vi "Reset Manual Layout.vi"(8 "error in":errorcluster, 11 "Base Software in":refnum<class "Base Software.lvclass">) -> (0 "error out":errorcluster, 3 "Base Software out":refnum<class "Base Software.lvclass">)   [LabVIEW 2019, in "Base Software.lvlib" / "Main.lvlib" / "Base Software.lvclass"]
uses:
  Project/Base Software.lvclass
  Custom Controls/g_Identifiers.vi
  builds/Engine/Engine.lvlibp/Engine Messages/Reset Manual Layout Msg/Reset Manual Layout Msg.lvclass
  builds/Engine/Engine.lvlibp/Project/Engine.lvclass
  C:/Users/Public/Documents/Development/builds/Engine/Engine.lvlibp/Project/Engine.lvclass
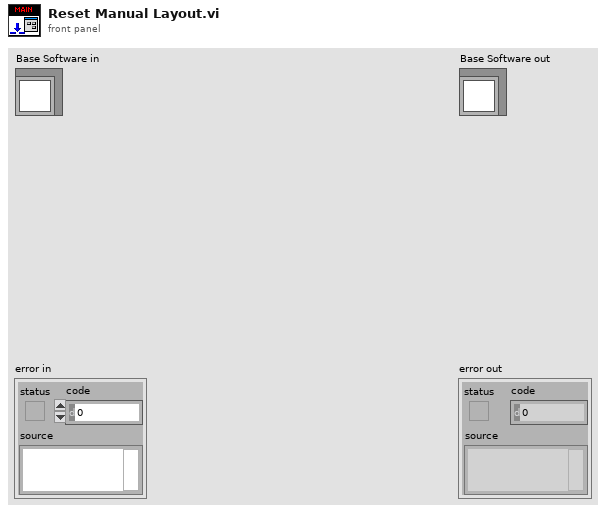
[diagram p1: front panel]
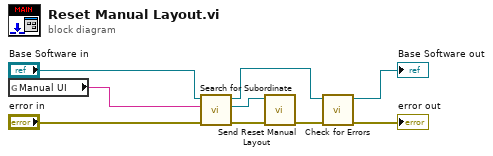
[diagram p0: block diagram]
diagram:
  n1 = global read "g_Identifiers.vi" "Manual UI"() -> (w7:string)
  n2 = call "Search for Subordinate.vi"("error in"="error in", "Identifier"=w7, "Base Software in"="Base Software in") -> ("error out"=w5:errorcluster, "Enqueuer"=w6:refnum<class "Message Enqueuer.lvclass">, "Base Software out"=w2:refnum<class "Base Software.lvclass">)  [unwired: 3 in, 3 out]
  n3 = call "Send Reset Manual Layout.vi"("error in (no error)"=w5, "Message Enqueuer"=w6) -> ("error out"=w1:errorcluster)  [unwired: 8 in, 1 out]
  n4 = call "Check for Errors.vi"("error in"=w1, "Engine in"=w2) -> ("error out"=→"error out":errorcluster, "Engine out"=→"Base Software out":refnum<class "Base Software.lvclass">)  [unwired: 8 in]
